vi "ITX2 Plot Commands.vi"(1 "X,Y Log":i32[](array[numeric]), 3 "input string":string="Display/R '#wave#'\nAppendToGraph '#wave#'\nLabel bottom \"#labelX#\"\nLabel left \"#labelY#\"\nModifyGraph rgb('#wave#')=(#r#,#g#,#b#)\n\\\\s('#wave#') #label#\nModifyGraph mirror(bottom)=1\nModifyGraph width=216\nModifyGraph height={Aspect,0.6}\nModifyGraph Log(bottom)=#bottomlog#\nModifyGraph Log(left)=#leftlog#", 4 "Plot labels":string[](array[string])=["time", "V", "V^2", "V^3"], 5 "X,Y Labels":string[](array[string])=["x label", "y label"], 6 "wavenames":string[](array[string])=["time.datatest.000005", "V.datatest.000005", "V^2.datatest.000005", "V^3.datatest.000005"]) -> (0 "result string":string="Display/R 'time.datatest.000005'\nAppendToGraph 'V.datatest.000005'\nAppendToGraph 'V^2.datatest.000005'\nAppendToGraph 'V^3.datatest.000005'\nLabel bottom \"x label\"\nLabel left \"y label\"\nModifyGraph rgb('time.datatest.000005')=(65280,0,0)\nModifyGraph rgb('V.datatest.000005')=(41984,65280,0)\nModifyGraph rgb('V^2.datatest.000005')=(0,65280,45568)\nModifyGraph rgb('V^3.datatest.000005')=(2048,0,65280)\nLegend/C/N=text0/J \"\\\\s('time.datatest.000005') time\\r\\\\s('V.datatest.000005') V\\r\\\\s('V^2.datatest.000005') V^2\\r\\\\s('V^3.datatest.000005') V^3\"\nModifyGraph mirror=1\nModifyGraph width=216\nModifyGraph height={Aspect,0.6}\nModifyGraph Log(bottom)=0\nModifyGraph Log(left)=0\n")   [LabVIEW 2020, in "Data.ITX.lvclass"]
uses:
  Data.ITX.lvclass
  graph_utilities/src/graph_utilities.lvclass
panel:
  # "Legend/C/N=text0/J \"\\\\s('y_test.000011Plot9') Plot 9\\r\\\\s('y_test.000011Plot8') Plot 8\""
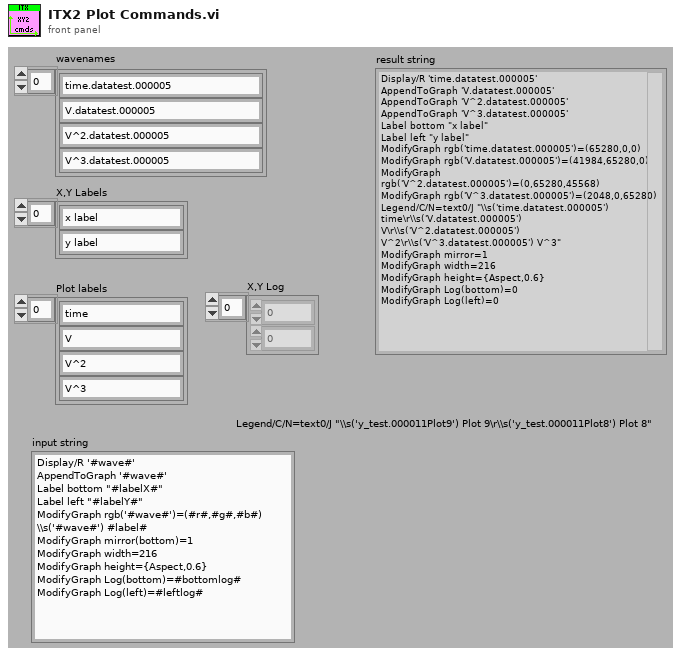
[diagram p1: front panel]
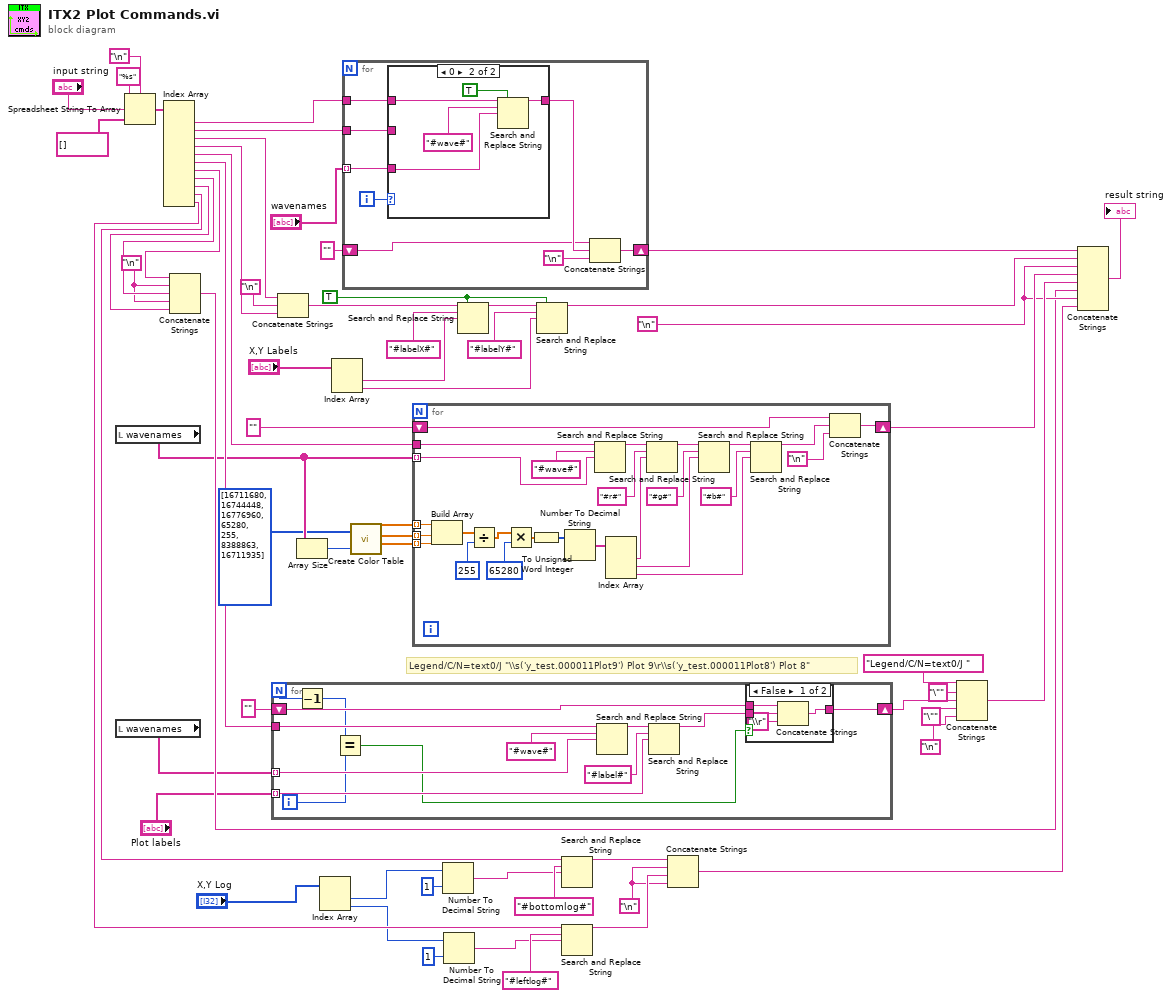
[diagram p0: block diagram]
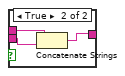
[diagram p2: hidden frame]
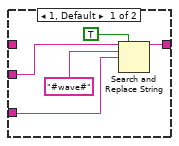
[diagram p3: hidden frame]
diagram:
  w17 = "\n"
  w26 = "\n"
  w25 = "\n"
  w47 = TRUE ("replace all? (F)")
  # "Legend/C/N=text0/J \"\\\\s('y_test.000011Plot9') Plot 9\\r\\\\s('y_test.000011Plot8') Plot 8\""
  n1 = local read "wavenames"() -> (w6:string[])
  n2 = local read "wavenames"() -> (w21:string[])
  n3 = Spreadsheet String To Array(delimiter (Tab)="\n", format string="%s", spreadsheet string="input string", array type (2D Dbl)=string[] []) -> (array=w56:string[])
  n4 = Index Array(array=w56) -> (element #1=w55:string, element #2=w54:string, element #3=w39:string, element #4=w40:string, element #5=w41:string, element #6=w37:string, element #7=w36:string, element #8=w35:string, element #9=w27:string, element #10=w15:string, element #11=w14:string)  [unwired: 11 in]
  n5 = Concatenate Strings(w36, w26, w35, w26, w27) -> (w24:string)
  n6 = for {
    N -> [w67]
    shift-right: [w68] -> w30
    shift-left: "" -> [w75]
    tunnel: "Plot labels" -> [w69] mode=indexing
    tunnel: w37 -> [w72]
    tunnel: w21 -> [w71] mode=indexing
    i -> [w65]
    n7 = Decrement(x=w67) -> (x-1=w66:i32)
    n8 = Equal?(x=w66, y=w65) -> (x = y?=w64:bool)
    n9 = Search and Replace String(input string=w72, search string="#wave#", replace string=w71) -> (result string=w76:string)  [unwired: 1 in, 7 out]
    n10 = Search and Replace String(input string=w76, search string="#label#", replace string=w69) -> (result string=w70:string)  [unwired: 1 in, 7 out]
    n11 = case shown="False" w64 {
      tunnel: w75 -> [w80 w82]
      tunnel: w70 -> [w79 w81]
      tunnel: [w78 w83] -> w68
      frame False {
        n12 = Concatenate Strings(w80, w79, "\\r" ("string")) -> (w78:string)
      }
      frame True {
        n13 = Concatenate Strings(w82, w81) -> (w83:string)
      }
    }
  }
  n14 = Concatenate Strings(w39, "\n", w40) -> (w52:string)
  n15 = Array Size(array=w6) -> (size(s)=w4:i32)
  n16 = Index Array(array="X,Y Log") -> (element #1=w8:i32, element #2=w7:i32)  [unwired: 2 in]
  n17 = Index Array(array="X,Y Labels") -> (element #1=w43:string, element #2=w42:string)  [unwired: 2 in]
  n18 = for {
    tunnel: "wavenames" -> [w89] mode=indexing
    tunnel: w55 -> [w91]
    tunnel: w54 -> [w90]
    shift-right: [w87] -> w60
    shift-left: "" -> [w84]
    i -> [w88]
    n19 = case shown="0" w88 {
      tunnel: w91 -> [_ w99]
      tunnel: w90 -> [w94 _]
      tunnel: w89 -> [w95 w100]
      tunnel: [w93 w98] -> w86
      frame 1, Default {
        n20 = Search and Replace String(replace all?=TRUE ("replace all? (F)"), input string=w94, search string="#wave#", replace string=w95) -> (result string=w93:string)  [unwired: 1 in, 6 out]
      }
      frame 0 {
        n21 = Search and Replace String(replace all?=TRUE ("replace all? (F)"), input string=w99, search string="#wave#", replace string=w100) -> (result string=w98:string)  [unwired: 1 in, 6 out]
      }
    }
    n22 = Concatenate Strings(w84, w86, "\n") -> (w87:string)
  }
  n23 = call "Create Color Table.vi"("Colors []"=u32[] [16711680, 16744448, 16776960, 65280, 255, 8388863, 16711935], "Size (256)"=w4) -> ("R []"=w1:dbl[], "G []"=w2:dbl[], "B []"=w3:dbl[])  [unwired: 1 out]
  n24 = for {
    tunnel: w41 -> [w120]
    tunnel: w6 -> [w105] mode=indexing
    shift-right: [w117] -> w45
    shift-left: "" -> [w116]
    tunnel: w3 -> [w104] mode=indexing
    tunnel: w2 -> [w103] mode=indexing
    tunnel: w1 -> [w102] mode=indexing
    n25 = Build Array(w102, w103, w104) -> (w127:dbl[])
    n26 = Divide(x=w127, y=255) -> (x/y=w123:dbl[])
    n27 = Multiply(x=w123, y=65280) -> (x*y=w124:dbl[])
    n28 = To Unsigned Word Integer(number=w124) -> (unsigned 16bit integer=w122:u16[])
    n29 = Number To Decimal String(number=w122) -> (decimal integer string=w110:string[])  [unwired: 1 out]
    n30 = Search and Replace String(input string=w120, search string="#wave#", replace string=w105) -> (result string=w121:string)  [unwired: 1 in, 7 out]
    n31 = Index Array(array=w110) -> (element #1=w109:string, element #2=w108:string, element #3=w107:string)  [unwired: 3 in]
    n32 = Search and Replace String(input string=w121, search string="#r#", replace string=w109) -> (result string=w119:string)  [unwired: 1 in, 7 out]
    n33 = Search and Replace String(input string=w119, search string="#g#", replace string=w108) -> (result string=w118:string)  [unwired: 1 in, 7 out]
    n34 = Search and Replace String(input string=w118, search string="#b#", replace string=w107) -> (result string=w114:string)  [unwired: 1 in, 7 out]
    n35 = Concatenate Strings(w116, w114, "\n") -> (w117:string)
  }
  n36 = Number To Decimal String(number=w8, width (-)=i16 1) -> (decimal integer string=w10:string)
  n37 = Number To Decimal String(number=w7, width (-)=i16 1) -> (decimal integer string=w11:string)
  n38 = Search and Replace String(replace all?=w47, input string=w52, search string="#labelX#", replace string=w43) -> (result string=w50:string)  [unwired: 1 in, 6 out]
  n39 = Search and Replace String(replace all?=w47, input string=w50, search string="#labelY#", replace string=w42) -> (result string=w38:string)  [unwired: 1 in, 6 out]
  n40 = Search and Replace String(input string=w15, search string="#bottomlog#", replace string=w10) -> (result string=w19:string)  [unwired: 1 in, 7 out]
  n41 = Search and Replace String(input string=w14, search string="#leftlog#", replace string=w11) -> (result string=w18:string)  [unwired: 1 in, 7 out]
  n42 = Concatenate Strings(w19, w17, w18, w17) -> (w16:string)
  n43 = Concatenate Strings("Legend/C/N=text0/J ", "\"" ("string"), w30, "\"" ("string"), "\n") -> (w32:string)
  n44 = Concatenate Strings(w60, w38, w25, w45, w32, w24, w25, w16) -> (→"result string":string)
